vi "Finish.vi"   [LabVIEW 2020]
doc: "This VI is called just before exiting. It is expected to close I/O refnum, save collected data, etc."
uses:
  mechanisms.ctl
  <vilib>/Rock Robotics/WPI/Utilities/WPI_GetSetVariantRefNum.vi
types:
  T1 = typedef "mechanisms.ctl" = string
  T2 = typedef "WPI_JoystickDevRef.ctl" = cluster{"Device":T3}
  T3 = typedef "WPI_JoystickDeviceEnum.ctl" = enum16{"USB 0", "USB 1", "USB 2", "USB 3", "USB 4", "USB 5"}
  T4 = typedef "WPI_MotorControlDeviceRef.ctl" = cluster{"DeviceStatus":errorcluster, "Type":T5, "PWM":cluster{"PWM Channel":T6, "DeadBand":T7}, "CAN":cluster{"Device Number":u8, "SetOutput VI Ref":variant, "GetOutput VI Ref":variant, "Enable VI Ref":variant, "Disable VI Ref":variant, "Data":variant}, "Invert":bool, "DIO PWM":cluster{"PWM \"Enable\" Channel":T6, "DIOChannel":T8, "PWM Rate":dbl}}
  T5 = typedef "WPI_MotorControlType.ctl" = enum16{"PWM", "CAN", "DIO PWM"}
  T6 = typedef "FPGA_DIOPWMChannel.ctl" = enum8{"PWM 0", "PWM 1", "PWM 2", "PWM 3", "PWM 4", "PWM 5", "PWM 6", "PWM 7", "PWM 8", "PWM 9", "PWM MXP 0", "PWM MXP 1", "PWM MXP 2", "PWM MXP 3", "PWM MXP 4", "PWM MXP 5", "PWM MXP 6", "PWM MXP 7", "PWM MXP 8", "PWM MXP 9", "Invalid"}
  T7 = typedef "WPI_PWMDeadband.ctl" = cluster{"Name":string, "maxPositivePwm":i32, "minPositivePwm":i32, "centerPwm":i32, "maxNegativePwm":i32, "minNegativePwm":i32, "angularRange":u16}
  T8 = typedef "FPGA_DIOChannel.ctl" = enum8{"DIO 0", "DIO 1", "DIO 2", "DIO 3", "DIO 4", "DIO 5", "DIO 6", "DIO 7", "DIO 8", "DIO 9", "DIO MXP 0", "DIO MXP 1", "DIO MXP 2", "DIO MXP 3", "DIO MXP 4", "DIO MXP 5", "DIO MXP 6", "DIO MXP 7", "DIO MXP 8", "DIO MXP 9", "DIO MXP 10", "DIO MXP 11", "DIO MXP 12", "DIO MXP 13", "DIO MXP 14", "DIO MXP 15", "SPI Port CS1", "SPI Port CS2", "SPI Port CS3", "SPI Port MISO", "SPI Port MOSI", "Invalid"}
  T9 = typedef "Color Sensor V3 DevRef.ctl" = cluster{"I2CDevRef":T10}
  T10 = typedef "WPI_I2CDevRef.ctl" = cluster{"DevStatus":errorcluster, "Device Address":u8, "Handle":i32, "I2C Bus":T11}
  T11 = typedef "i2c_bus.ctl" = enum16{"I2C On-Board", "I2C MXP", "Invalid"}
  T12 = typedef "WPI_CompressorDevRef.ctl" = cluster{"DevStatus":errorcluster, "Pneumatics Control Module":u8}
  T13 = typedef "WPI_SolenoidDevRef.ctl" = cluster{"DevStatus":errorcluster, "Pneumatics Control Module":u8, "Forward Solenoid Channel":T14, "Reverse Solenoid Channel":T14}
  T14 = typedef "WPI_SolenoidChannel.ctl" = enum8{"Solenoid 0", "Solenoid 1", "Solenoid 2", "Solenoid 3", "Solenoid 4", "Solenoid 5", "Solenoid 6", "Solenoid 7", "Solenoid 8", "Solenoid 9", "Solenoid 10", "Solenoid 11", "Solenoid 12", "Solenoid 13", "Solenoid 14", "Solenoid 15", "Invalid"}
  T15 = typedef "WPI_SwitchDevRef.ctl" = cluster{"DevStatus":errorcluster, "DIO Channel":T8, "CntIndex":T16, "Normally Closed":bool}
  T16 = typedef "FPGA_CounterCtrSystemIndex.ctl" = enum8{"Ctr 0", "Ctr 1", "Ctr 2", "Ctr 3", "Ctr 4", "Ctr 5", "Ctr 6", "Ctr 7", "Invalid"}
  T17 = typedef "WPI_DigitalInputDevRef.ctl" = cluster{"DevStatus":errorcluster, "DIO Channel":T8}
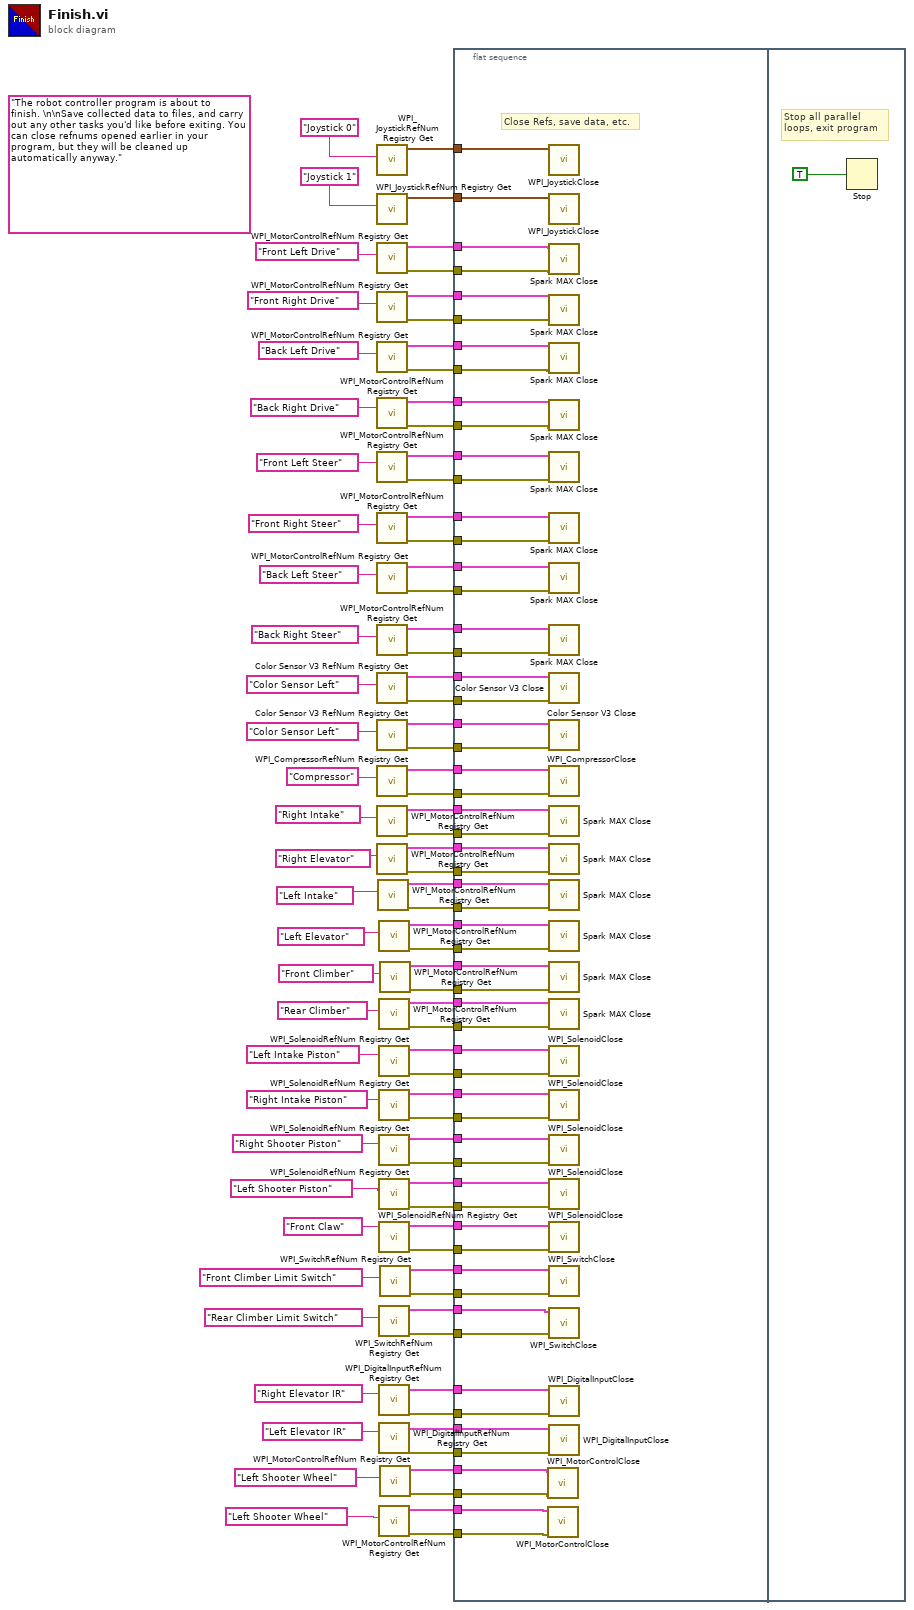
[diagram p0: block diagram]
diagram:
  (unwired) "The robot controller program is about to finish. \n\nSave collected data to files, and carry out any other tasks you'd like before exiting. You can close refnums opened earlier in your program, but they will be cleaned up automatically anyway."
  n1 = call <vilib>:"WPI_JoystickRefNum Registry Get.vi"("refnum name"="Joystick 0") -> ("JoystickDevRef"=w87:T2)  [unwired: 1 in, 9 out]
  n2 = call <vilib>:"WPI_JoystickRefNum Registry Get.vi"("refnum name"="Joystick 1") -> ("JoystickDevRef"=w85:T2)  [unwired: 1 in, 9 out]
  n3 = call <vilib>:"WPI_MotorControlRefNum Registry Get.vi"("refnum name"="Front Left Drive" ("Motor References")) -> ("error out"=w83:errorcluster, "MotorControlDevRef"=w84:T4)  [unwired: 9 in]
  n4 = call <vilib>:"WPI_MotorControlRefNum Registry Get.vi"("refnum name"="Front Right Drive" ("Motor References")) -> ("error out"=w81:errorcluster, "MotorControlDevRef"=w82:T4)  [unwired: 9 in]
  n5 = call <vilib>:"WPI_MotorControlRefNum Registry Get.vi"("refnum name"="Back Left Drive" ("Motor References")) -> ("error out"=w79:errorcluster, "MotorControlDevRef"=w80:T4)  [unwired: 9 in]
  n6 = call <vilib>:"WPI_MotorControlRefNum Registry Get.vi"("refnum name"="Back Right Drive" ("Motor References")) -> ("error out"=w77:errorcluster, "MotorControlDevRef"=w78:T4)  [unwired: 9 in]
  n7 = call <vilib>:"WPI_MotorControlRefNum Registry Get.vi"("refnum name"="Front Left Steer" ("Motor References")) -> ("error out"=w75:errorcluster, "MotorControlDevRef"=w76:T4)  [unwired: 9 in]
  n8 = call <vilib>:"WPI_MotorControlRefNum Registry Get.vi"("refnum name"="Front Right Steer" ("Motor References")) -> ("error out"=w73:errorcluster, "MotorControlDevRef"=w74:T4)  [unwired: 9 in]
  n9 = call <vilib>:"WPI_MotorControlRefNum Registry Get.vi"("refnum name"="Back Left Steer" ("Motor References")) -> ("error out"=w71:errorcluster, "MotorControlDevRef"=w72:T4)  [unwired: 9 in]
  n10 = call <vilib>:"WPI_MotorControlRefNum Registry Get.vi"("refnum name"="Back Right Steer" ("Motor References")) -> ("error out"=w69:errorcluster, "MotorControlDevRef"=w70:T4)  [unwired: 9 in]
  n11 = call <vilib>:"Color Sensor V3 RefNum Registry Get.vi"("refnum name"=T1 "Color Sensor Left" ("Mechanism")) -> ("error out"=w64:errorcluster, "ColorSensorDevRef"=w65:T9)  [unwired: 9 in]
  n12 = call <vilib>:"Color Sensor V3 RefNum Registry Get.vi"("refnum name"=T1 "Color Sensor Left" ("Mechanism")) -> ("error out"=w60:errorcluster, "ColorSensorDevRef"=w63:T9)  [unwired: 9 in]
  n13 = call <vilib>:"WPI_CompressorRefNum Registry Get.vi"("refnum name"="Compressor") -> ("error out"=w61:errorcluster, "CompressorDevRef"=w62:T12)  [unwired: 9 in]
  n14 = call <vilib>:"WPI_MotorControlRefNum Registry Get.vi"("refnum name"=T1 "Right Intake" ("Mechanism")) -> ("error out"=w52:errorcluster, "MotorControlDevRef"=w53:T4)  [unwired: 9 in]
  n15 = call <vilib>:"WPI_MotorControlRefNum Registry Get.vi"("refnum name"=T1 "Right Elevator" ("Mechanism")) -> ("error out"=w50:errorcluster, "MotorControlDevRef"=w51:T4)  [unwired: 9 in]
  n16 = call <vilib>:"WPI_MotorControlRefNum Registry Get.vi"("refnum name"=T1 "Left Intake" ("Mechanism")) -> ("error out"=w48:errorcluster, "MotorControlDevRef"=w49:T4)  [unwired: 9 in]
  n17 = call <vilib>:"WPI_MotorControlRefNum Registry Get.vi"("refnum name"=T1 "Left Elevator" ("Mechanism")) -> ("error out"=w46:errorcluster, "MotorControlDevRef"=w47:T4)  [unwired: 9 in]
  n18 = call <vilib>:"WPI_MotorControlRefNum Registry Get.vi"("refnum name"=T1 "Rear Climber" ("Mechanism")) -> ("error out"=w42:errorcluster, "MotorControlDevRef"=w43:T4)  [unwired: 9 in]
  n19 = call <vilib>:"WPI_SolenoidRefNum Registry Get.vi"("refnum name"=T1 "Left Intake Piston" ("Mechanism")) -> ("error out"=w37:errorcluster, "SolenoidDevRef"=w38:T13)  [unwired: 9 in]
  n20 = call <vilib>:"WPI_SolenoidRefNum Registry Get.vi"("refnum name"=T1 "Right Intake Piston" ("Mechanism")) -> ("error out"=w35:errorcluster, "SolenoidDevRef"=w36:T13)  [unwired: 9 in]
  n21 = call <vilib>:"WPI_SolenoidRefNum Registry Get.vi"("refnum name"=T1 "Right Shooter Piston" ("Mechanisms")) -> ("error out"=w33:errorcluster, "SolenoidDevRef"=w34:T13)  [unwired: 9 in]
  n22 = call <vilib>:"WPI_SolenoidRefNum Registry Get.vi"("refnum name"=T1 "Left Shooter Piston" ("Mechanisms")) -> ("error out"=w31:errorcluster, "SolenoidDevRef"=w32:T13)  [unwired: 9 in]
  n23 = call <vilib>:"WPI_SolenoidRefNum Registry Get.vi"("refnum name"=T1 "Front Claw" ("Mechanism")) -> ("error out"=w29:errorcluster, "SolenoidDevRef"=w30:T13)  [unwired: 9 in]
  n24 = call <vilib>:"WPI_SwitchRefNum Registry Get.vi"("refnum name"=T1 "Rear Climber Limit Switch" ("Mechanisms")) -> ("error out"=w13:errorcluster, "SwitchDevRef"=w15:T15)  [unwired: 9 in]
  n25 = call <vilib>:"WPI_DigitalInputRefNum Registry Get.vi"("refnum name"=T1 "Right Elevator IR" ("Mechanisms")) -> ("error out"=w9:errorcluster, "DigitalInputDevRef"=w10:T17)  [unwired: 9 in]
  n26 = call <vilib>:"WPI_DigitalInputRefNum Registry Get.vi"("refnum name"=T1 "Left Elevator IR" ("Mechanisms")) -> ("error out"=w7:errorcluster, "DigitalInputDevRef"=w8:T17)  [unwired: 9 in]
  n27 = call <vilib>:"WPI_MotorControlRefNum Registry Get.vi"("refnum name"=T1 "Left Shooter Wheel" ("Mechanisms")) -> ("error out"=w1:errorcluster, "MotorControlDevRef"=w2:T4)  [unwired: 9 in]
  n28 = call <vilib>:"WPI_MotorControlRefNum Registry Get.vi"("refnum name"=T1 "Front Climber" ("Mechanism")) -> ("error out"=w44:errorcluster, "MotorControlDevRef"=w45:T4)  [unwired: 9 in]
  n29 = call <vilib>:"WPI_SwitchRefNum Registry Get.vi"("refnum name"=T1 "Front Climber Limit Switch" ("Mechanisms")) -> ("error out"=w14:errorcluster, "SwitchDevRef"=w16:T15)  [unwired: 9 in]
  n30 = call <vilib>:"WPI_MotorControlRefNum Registry Get.vi"("refnum name"=T1 "Left Shooter Wheel" ("Mechanisms")) -> ("error out"=w3:errorcluster, "MotorControlDevRef"=w4:T4)  [unwired: 9 in]
  n31 = flat-sequence {
    tunnel: w87 -> [w146]
    tunnel: w85 -> [w145]
    tunnel: w84 -> [w144]
    tunnel: w83 -> [w143]
    tunnel: w82 -> [w142]
    tunnel: w81 -> [w141]
    tunnel: w80 -> [w140]
    tunnel: w79 -> [w139]
    tunnel: w78 -> [w138]
    tunnel: w77 -> [w137]
    tunnel: w76 -> [w123]
    tunnel: w75 -> [w124]
    tunnel: w74 -> [w125]
    tunnel: w73 -> [w126]
    tunnel: w72 -> [w127]
    tunnel: w71 -> [w128]
    tunnel: w70 -> [w130]
    tunnel: w69 -> [w129]
    tunnel: w65 -> [w136]
    tunnel: w64 -> [w135]
    tunnel: w63 -> [w134]
    tunnel: w62 -> [w133]
    tunnel: w61 -> [w132]
    tunnel: w60 -> [w131]
    tunnel: w53 -> [w122]
    tunnel: w52 -> [w121]
    tunnel: w51 -> [w120]
    tunnel: w50 -> [w119]
    tunnel: w49 -> [w118]
    tunnel: w48 -> [w117]
    tunnel: w47 -> [w116]
    tunnel: w46 -> [w115]
    tunnel: w45 -> [w114]
    tunnel: w44 -> [w113]
    tunnel: w43 -> [w112]
    tunnel: w42 -> [w111]
    tunnel: w38 -> [w110]
    tunnel: w37 -> [w109]
    tunnel: w36 -> [w108]
    tunnel: w35 -> [w107]
    tunnel: w34 -> [w106]
    tunnel: w33 -> [w105]
    tunnel: w32 -> [w104]
    tunnel: w31 -> [w103]
    tunnel: w30 -> [w102]
    tunnel: w29 -> [w101]
    tunnel: w16 -> [w100]
    tunnel: w15 -> [w99]
    tunnel: w14 -> [w98]
    tunnel: w13 -> [w97]
    tunnel: w10 -> [w96]
    tunnel: w9 -> [w95]
    tunnel: w8 -> [w94]
    tunnel: w7 -> [w93]
    tunnel: w4 -> [w92]
    tunnel: w3 -> [w91]
    tunnel: w2 -> [w90]
    tunnel: w1 -> [w89]
    frame #0 {
      # "Close Refs, save data, etc."
      n32 = call <vilib>:"WPI_MotorControlClose.vi"("error in"=w91, "MotorControlDevRef"=w92) -> ()  [unwired: 9 in, 1 out]
      n33 = call <vilib>:"WPI_MotorControlClose.vi"("error in"=w89, "MotorControlDevRef"=w90) -> ()  [unwired: 9 in, 1 out]
      n34 = call <vilib>:"WPI_JoystickClose.vi"("JoystickDevRef"=w146) -> ()  [unwired: 11 out]
      n35 = call <vilib>:"WPI_JoystickClose.vi"("JoystickDevRef"=w145) -> ()  [unwired: 11 out]
      n36 = call <vilib>:"Spark MAX Close.vi"("error in"=w143, "MotorControlDeviceRef"=w144) -> ()  [unwired: 9 in, 1 out]
      n37 = call <vilib>:"Spark MAX Close.vi"("error in"=w141, "MotorControlDeviceRef"=w142) -> ()  [unwired: 9 in, 1 out]
      n38 = call <vilib>:"Spark MAX Close.vi"("error in"=w139, "MotorControlDeviceRef"=w140) -> ()  [unwired: 9 in, 1 out]
      n39 = call <vilib>:"Spark MAX Close.vi"("error in"=w137, "MotorControlDeviceRef"=w138) -> ()  [unwired: 9 in, 1 out]
      n40 = call <vilib>:"Spark MAX Close.vi"("error in"=w124, "MotorControlDeviceRef"=w123) -> ()  [unwired: 9 in, 1 out]
      n41 = call <vilib>:"Spark MAX Close.vi"("error in"=w126, "MotorControlDeviceRef"=w125) -> ()  [unwired: 9 in, 1 out]
      n42 = call <vilib>:"Spark MAX Close.vi"("error in"=w128, "MotorControlDeviceRef"=w127) -> ()  [unwired: 9 in, 1 out]
      n43 = call <vilib>:"Spark MAX Close.vi"("error in"=w129, "MotorControlDeviceRef"=w130) -> ()  [unwired: 9 in, 1 out]
      n44 = call <vilib>:"Color Sensor V3 Close.vi"("error in (no error)"=w135, "ColorSensorDevRef in"=w136) -> ()  [unwired: 9 in, 1 out]
      n45 = call <vilib>:"Color Sensor V3 Close.vi"("error in (no error)"=w131, "ColorSensorDevRef in"=w134) -> ()  [unwired: 9 in, 1 out]
      n46 = call <vilib>:"WPI_CompressorClose.vi"("error in (no error)"=w132, "CompressorDevRef"=w133) -> ()  [unwired: 9 in, 1 out]
      n47 = call <vilib>:"Spark MAX Close.vi"("error in"=w121, "MotorControlDeviceRef"=w122) -> ()  [unwired: 9 in, 1 out]
      n48 = call <vilib>:"Spark MAX Close.vi"("error in"=w119, "MotorControlDeviceRef"=w120) -> ()  [unwired: 9 in, 1 out]
      n49 = call <vilib>:"Spark MAX Close.vi"("error in"=w117, "MotorControlDeviceRef"=w118) -> ()  [unwired: 9 in, 1 out]
      n50 = call <vilib>:"Spark MAX Close.vi"("error in"=w115, "MotorControlDeviceRef"=w116) -> ()  [unwired: 9 in, 1 out]
      n51 = call <vilib>:"Spark MAX Close.vi"("error in"=w113, "MotorControlDeviceRef"=w114) -> ()  [unwired: 9 in, 1 out]
      n52 = call <vilib>:"Spark MAX Close.vi"("error in"=w111, "MotorControlDeviceRef"=w112) -> ()  [unwired: 9 in, 1 out]
      n53 = call <vilib>:"WPI_SolenoidClose.vi"("error in (no error)"=w109, "SolenoidDevRef"=w110) -> ()  [unwired: 9 in, 1 out]
      n54 = call <vilib>:"WPI_SolenoidClose.vi"("error in (no error)"=w107, "SolenoidDevRef"=w108) -> ()  [unwired: 9 in, 1 out]
      n55 = call <vilib>:"WPI_SolenoidClose.vi"("error in (no error)"=w105, "SolenoidDevRef"=w106) -> ()  [unwired: 9 in, 1 out]
      n56 = call <vilib>:"WPI_SolenoidClose.vi"("error in (no error)"=w103, "SolenoidDevRef"=w104) -> ()  [unwired: 9 in, 1 out]
      n57 = call <vilib>:"WPI_SolenoidClose.vi"("error in (no error)"=w101, "SolenoidDevRef"=w102) -> ()  [unwired: 9 in, 1 out]
      n58 = call <vilib>:"WPI_SwitchClose.vi"("error in (no error)"=w98, "SwitchDevRef"=w100) -> ()  [unwired: 9 in, 1 out]
      n59 = call <vilib>:"WPI_SwitchClose.vi"("error in (no error)"=w97, "SwitchDevRef"=w99) -> ()  [unwired: 9 in, 1 out]
      n60 = call <vilib>:"WPI_DigitalInputClose.vi"("error in (no error)"=w95, "DigitalInputDevRef"=w96) -> ()  [unwired: 9 in, 1 out]
      n61 = call <vilib>:"WPI_DigitalInputClose.vi"("error in (no error)"=w93, "DigitalInputDevRef"=w94) -> ()  [unwired: 9 in, 1 out]
    }
    frame #1 {
      # "Stop all parallel\nloops, exit program"
      n62 = Stop(stop? (T)=TRUE ("Quit")) -> ()
    }
  }
